vi "Database Main.vi"(11 "Application.lvclass":refnum<class "Application.lvclass">) -> (2 "Stats":string[][](table) caption="Result Set (from first statement with results)", 3 "Games":string[][](table) caption="Result Set (from first statement with results)")   [LabVIEW 2021, in "Application.lvclass"]
uses:
  Application.lvclass
  <vilib>/drjdpowell/SQLite Library/SQL Connection/Connection.lvclass
  Globales Snake.vi
  <vilib>/drjdpowell/SQLite Library/SQL Connection/Execute SQL.vi
  <vilib>/drjdpowell/SQLite Library/SQL Connection/Open (path).vi
  <vilib>/drjdpowell/SQLite Library/SQL Connection/Execute SQL (No results).vi
  Board Game_class/Board Game.lvclass
panel:
  in  "error in (no error)":errorcluster
  out "error out":errorcluster
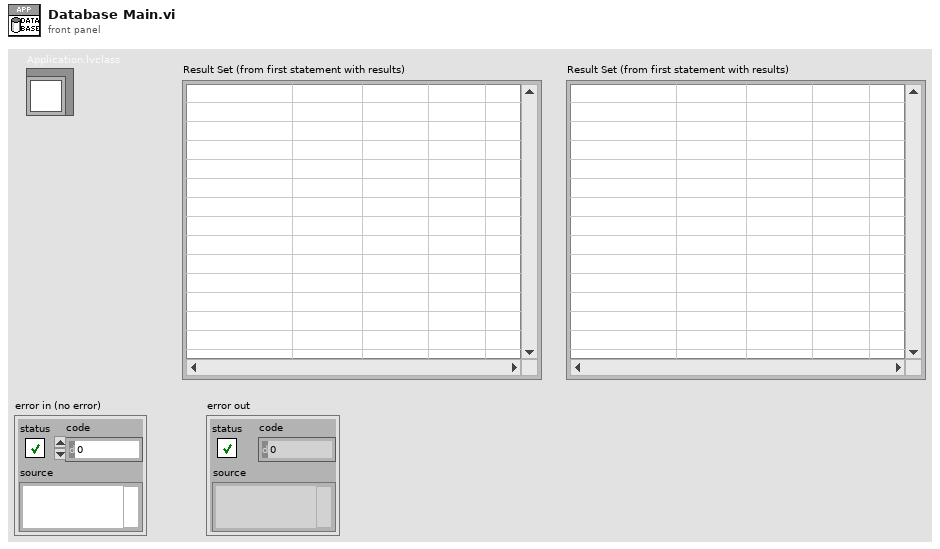
[diagram p1: front panel]
types:
  T1 = enum16{"New or existing", "Existing", "Read only"}
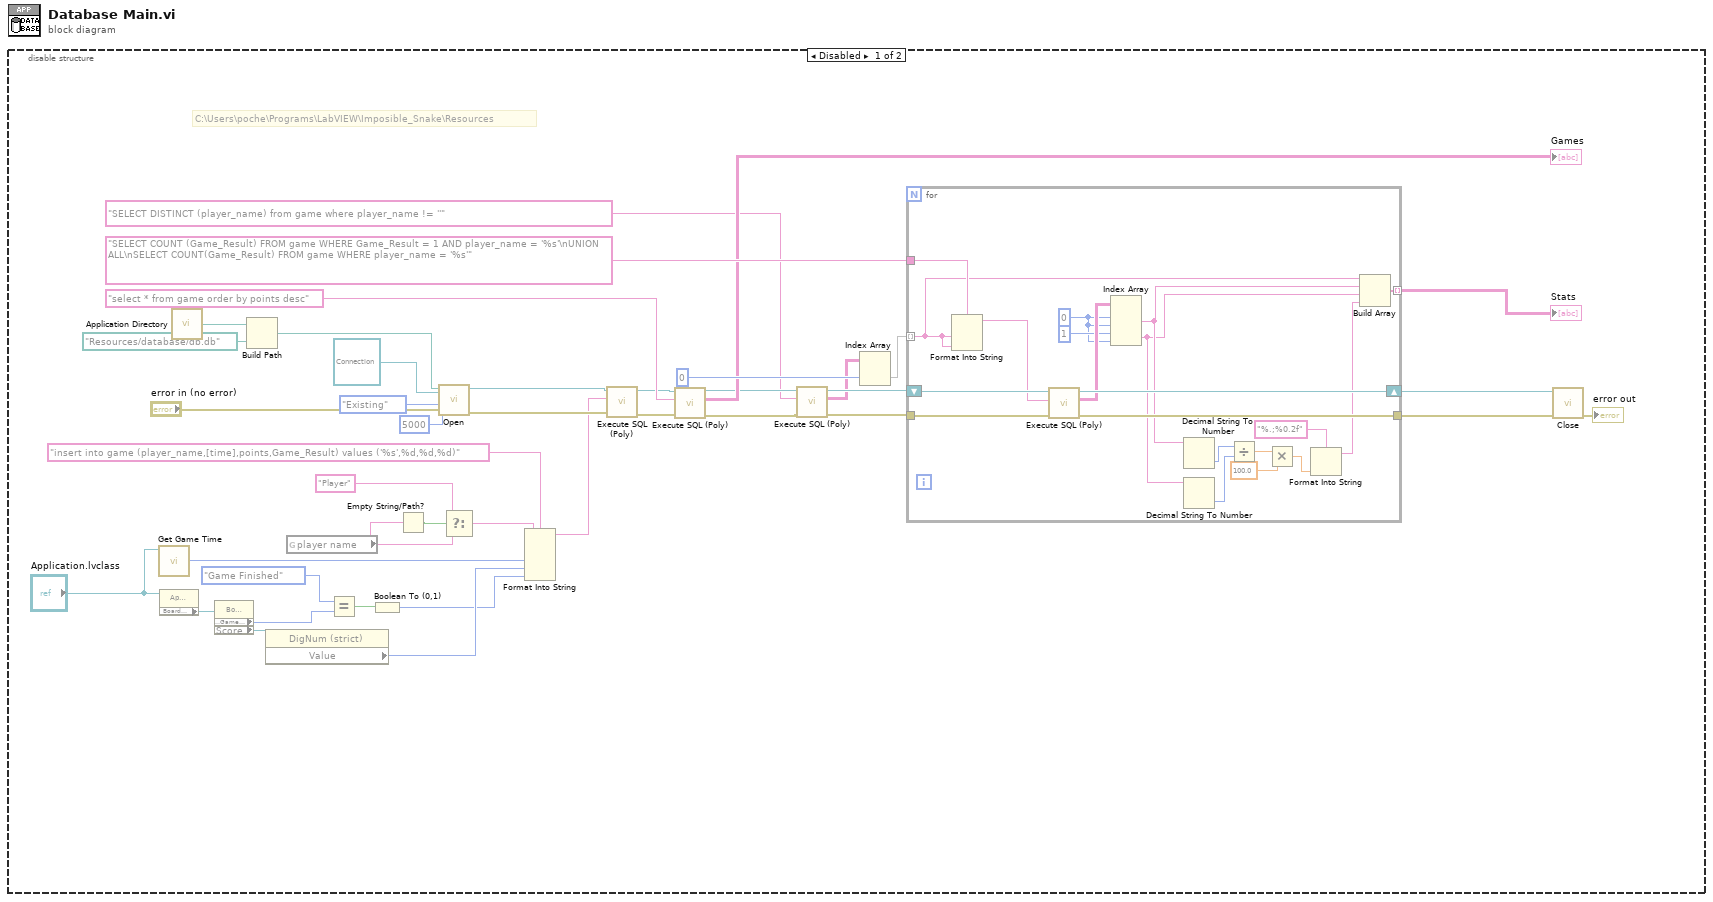
[diagram p0: block diagram]
diagram:
  n1 = disable-structure shown="Disabled" {
    frame Disabled {
      # "C:\\Users\\poche\\Programs\\LabVIEW\\Imposible_Snake\\Resources"
      n2 = call "Get Game Time.vi"("Application in"="Application.lvclass") -> ("Elapsed"=w26:u32)  [unwired: 8 in, 2 out]
      n3 = property class="Application.lvclass"(reference="Application.lvclass") -> ("Board Game"=w24:refnum<class "Board Game.lvclass">)  [unwired: 1 in, 2 out]
      n4 = call <vilib>:"Application Directory.vi"() -> ("Application Directory"=w35:path)
      n5 = property class="Board Game"(reference=w24) -> ("dataAccess:Game Result"=w17:enum16{"Game Over", "Game Finished"}, "Score"=w23:refnum<vi>)  [unwired: 1 in, 2 out]
      n6 = Build Path(base path=w35, name or relative path=path "Resources/database/db.db") -> (appended path=w33:path)
      n7 = property class="DigNum (strict)"(reference=w23) -> ("Value"=w22:u16)  [unwired: 1 in, 2 out]
      n8 = global read "Globales Snake.vi" "player name"() -> (w18:string)
      n9 = Equal?(x=enum16{"Game Over", "Game Finished"}."Game Finished", y=w17) -> (x = y?=w15:bool)
      n10 = Boolean To (0,1)(Boolean=w15) -> (0, 1=w14:i16)
      n11 = Empty String/Path?(string/path=w18) -> (empty?=w20:bool)
      n12 = call-poly <vilib>:"Open.vi"("SQLite Connection type"=refnum<class "Connection.lvclass"> refnum, "error in (no error)"="error in (no error)", "File Option"=T1."Existing", "busy timeout (ms)"=5000, "db file"=w33) -> ("error out"=w32:errorcluster, "SQLite Connection"=w30:refnum<class "Connection.lvclass">)  [unwired: 5 in]
      n13 = Select(t="Player" ("player name"), s=w20, f=w18) -> (s? t:f=w21:string)
      n14 = Format Into String(format string="insert into game (player_name,[time],points,Game_Result) values ('%s',%d,%d,%d)" ("SQL"), w21, w26, w22, w14) -> (resulting string=w28:string)  [unwired: 2 in, 1 out]
      n15 = call-poly <vilib>:"Execute SQL (Poly).vi"("error in (no error)"=w32, "SQL"=w28, "SQLite Connection in"=w30) -> ("error out"=w31:errorcluster, "SQLite Connection"=w29:refnum<class "Connection.lvclass">)  [unwired: 7 in]
      n16 = call-poly <vilib>:"Execute SQL (Poly).vi"("error in (no error)"=w31, "SQL"="select * from game order by points desc", "SQLite Connection in"=w29) -> ("error out"=w9:errorcluster, "Result Set"=→"Games":string[][], "SQLite Connection"=w8:refnum<class "Connection.lvclass">)  [unwired: 5 in, 1 out]
      n17 = call-poly <vilib>:"Execute SQL (Poly).vi"("error in (no error)"=w9, "SQL"="SELECT DISTINCT (player_name) from game where player_name != ''", "SQLite Connection in"=w8) -> ("error out"=w7:errorcluster, "Result Set"=w5:string[][], "SQLite Connection"=w6:refnum<class "Connection.lvclass">)  [unwired: 5 in, 1 out]
      n18 = Index Array(array=w5, index (col)=0 ("disabled index (col)")) -> (element=w12:string[])  [unwired: 1 in]
      n19 = for {
        shift-right: [w60] -> w2
        shift-left: w6 -> [w61]
        tunnel: w7 -> [w59]
        tunnel: [w58] -> w3
        tunnel: w12 -> [w54] mode=indexing
        tunnel: "SELECT COUNT (Game_Result) FROM game WHERE Game_Result = 1 AND player_name = '%s'\nUNION ALL\nSELECT COUNT(Game_Result) FROM game WHERE player_name = '%s'" ("SQL") -> [w57]
        tunnel: [w45] -> w1 mode=indexing
        w52 = 0 ("index (row)")
        n20 = Format Into String(format string=w57, w54, w54) -> (resulting string=w56:string)  [unwired: 2 in, 1 out]
        n21 = call-poly <vilib>:"Execute SQL (Poly).vi"("error in (no error)"=w59, "SQL"=w56, "SQLite Connection in"=w61) -> ("error out"=w58:errorcluster, "Result Set"=w55:string[][], "SQLite Connection"=w60:refnum<class "Connection.lvclass">)  [unwired: 5 in, 1 out]
        n22 = Index Array(array=w55, index (row) #1=w52, index (col) #1=w52, index (row) #2=1 ("index (row)"), index (col) #2=w52) -> (element #1=w44:string, element #2=w43:string)
        n23 = Decimal String To Number(string=w44) -> (number=w42:i32)  [unwired: 2 in, 1 out]
        n24 = Decimal String To Number(string=w43) -> (number=w51:i32)  [unwired: 2 in, 1 out]
        n25 = Divide(x=w42, y=w51) -> (x/y=w50:dbl)
        n26 = Multiply(x=w50, y=100.0) -> (x*y=w48:dbl)
        n27 = Format Into String(format string="%.;%0.2f", w48) -> (resulting string=w46:string)  [unwired: 2 in, 1 out]
        n28 = Build Array(w54, w44, w43, w46) -> (w45:string[])
      }
      "Stats" <- w1
      n29 = call-dynamic "Close.vi"("error in (no error)"=w3, "SQLite Connection in"=w2) -> ("error out"=→"error out":errorcluster)  [unwired: 9 in]
    }
    frame Enabled {
    }
  }
